vi "(Sub) Save.vi"(0 "IN Path":path, 2 "C Limit / Voltage":dbl[](array[numeric]), 3 "G1. V":dbl, 4 "G2. V":dbl, 5 "error in (no error)":errorcluster caption="에러 입력(에러 없음)", 6 "State":enum16{"Open", "Header Make", "Save", "Close"}(ring), 7 "G3. V":dbl, 8 "G1. Info":string, 9 "G1. A":dbl, 10 "G2. Info":string, 11 "G2. A":dbl, 12 "G3. Info":string, 13 "G3. A":dbl) -> (14 "Save Path":path, 19 "error out":errorcluster caption="에러 출력")   [LabVIEW 2017]
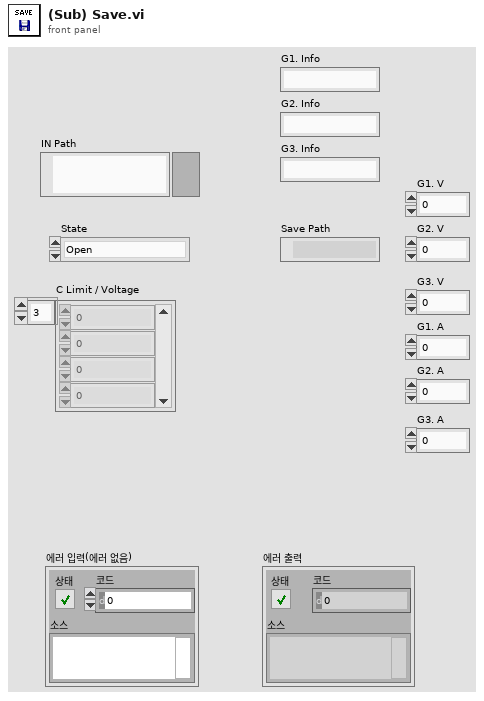
[diagram p1: front panel]
types:
  T1 = enum16{"open", "replace", "create", "open or create", "replace or create", "replace or create with confirmation"}
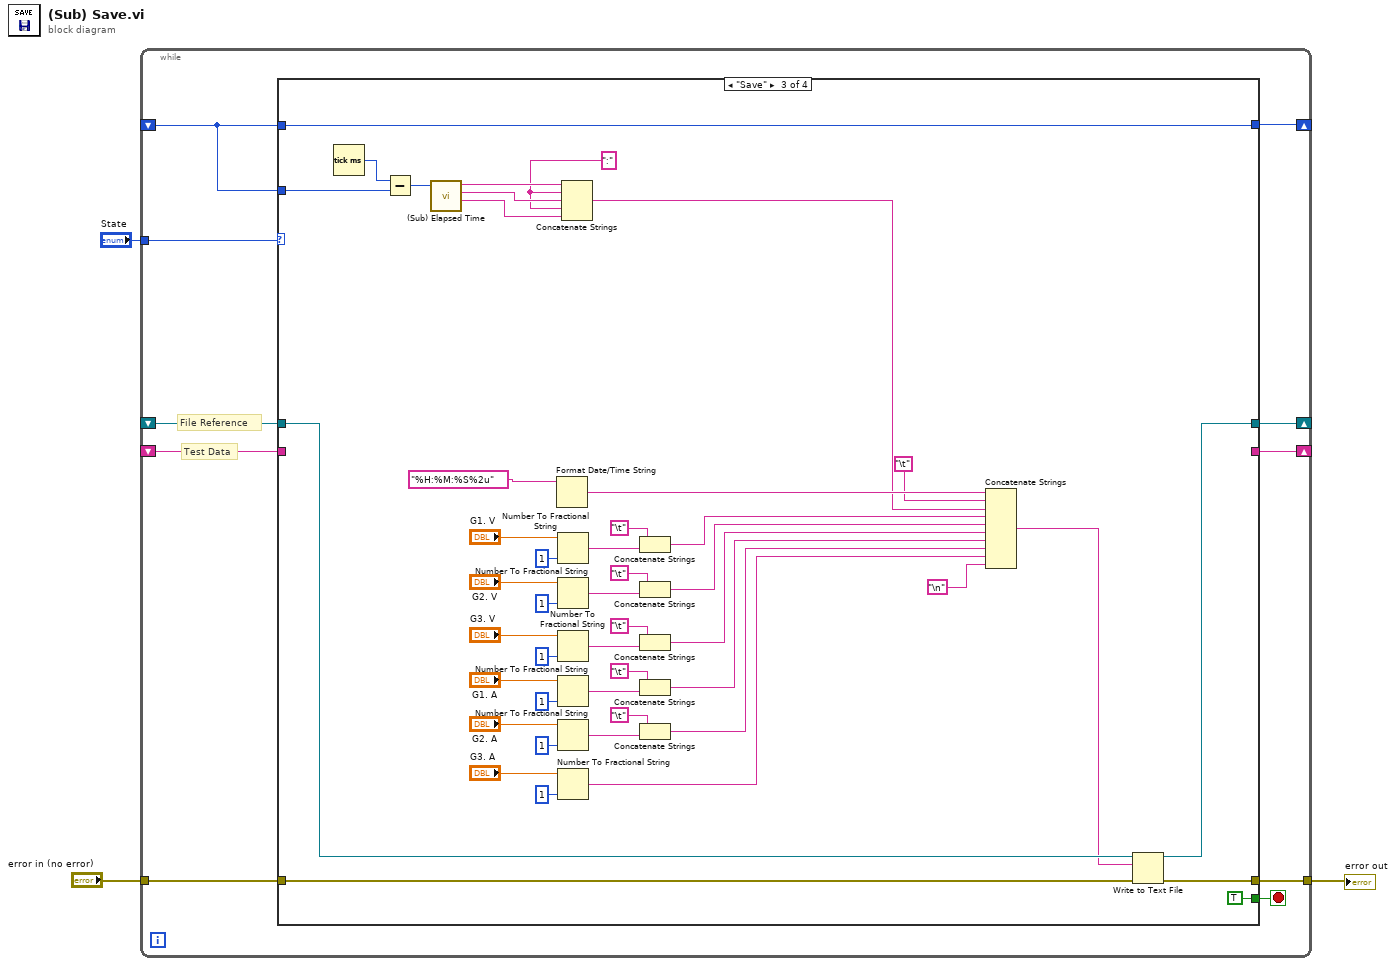
[diagram p0: block diagram]
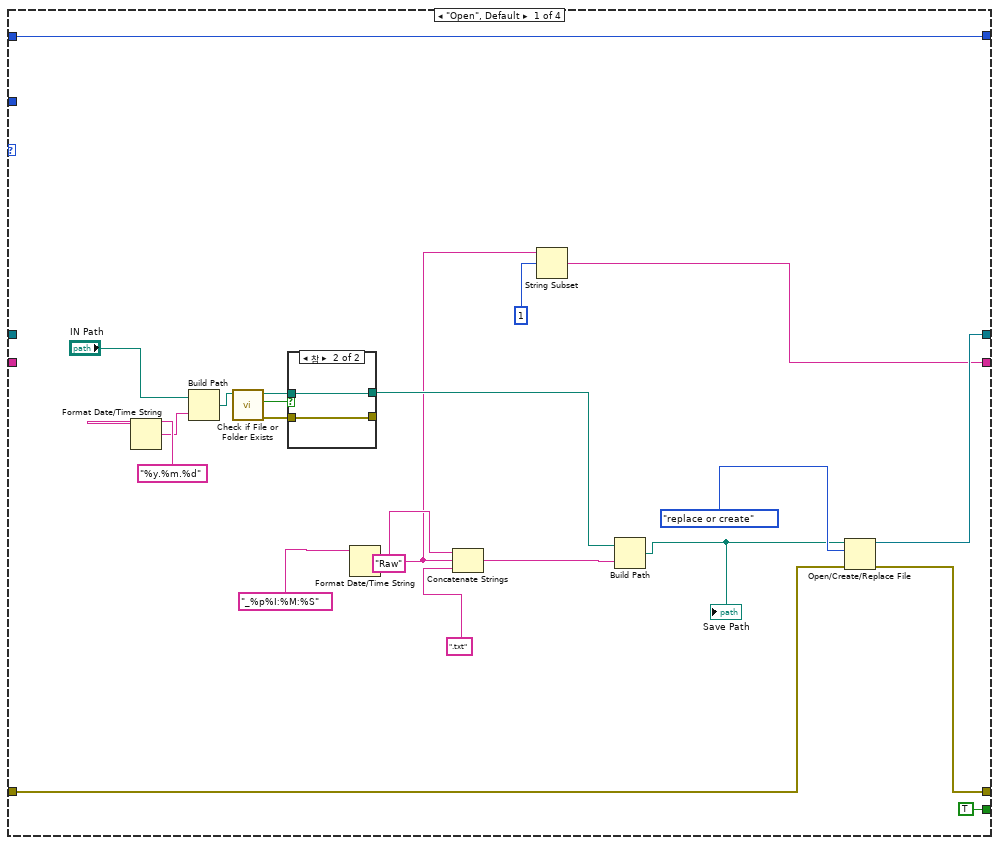
[diagram p2: hidden frame]
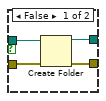
[diagram p3: hidden frame]
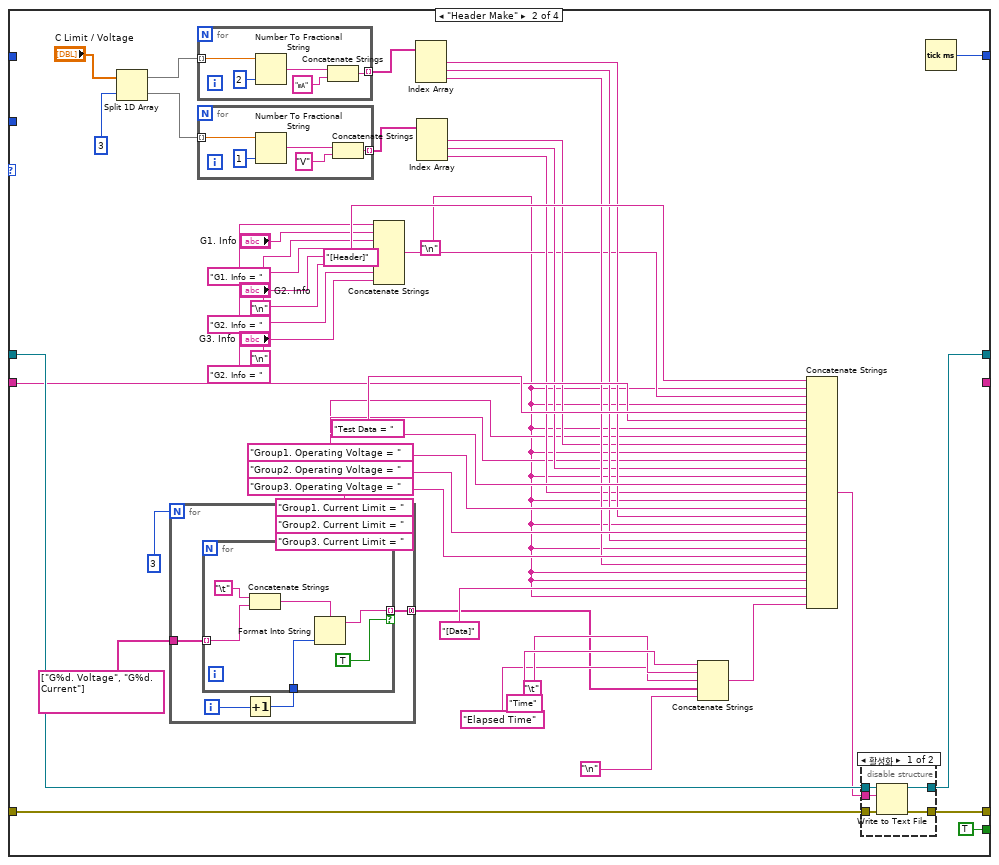
[diagram p4: hidden frame]
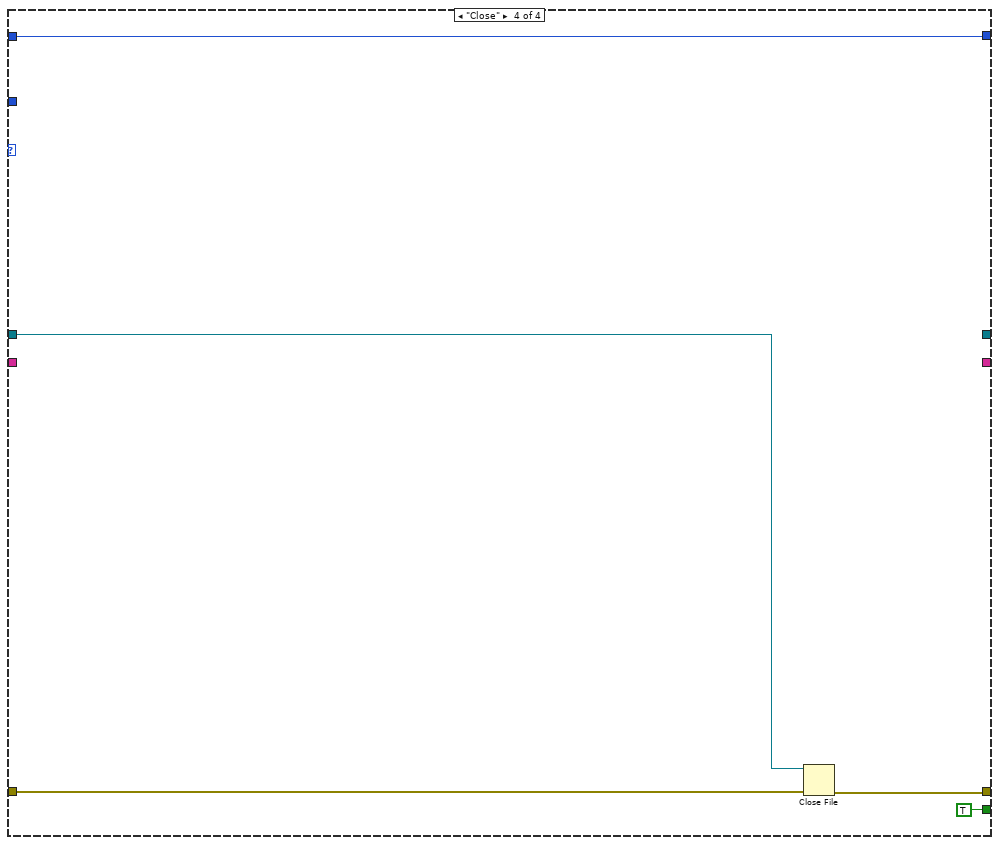
[diagram p6: hidden frame]
diagram:
  n1 = while {
    tunnel: [w10] -> w2
    tunnel: "error in (no error)" -> [w13]
    shift-right: [w11] -> _
    shift-left: _ -> [w12]
    shift-right: [w9] -> _
    shift-left: _ -> [w8]
    shift-right: [w6] -> _
    shift-left: _ -> [w5]
    tunnel: "State" -> [w4]
    stop <- w7 stop-if-true
    # "Test Data"
    # "File Reference"
    n2 = case shown="\"Save\"" w4 {
      tunnel: w13 -> [w30 w88 w160 w164]
      tunnel: w12 -> [_ w81 w157 w163]
      tunnel: [w33 w80 w154 _] -> w11
      tunnel: [w32 w87 w159 w165] -> w10
      tunnel: [w14 _ _ _] -> w9
      tunnel: w8 -> [_ w78 _ _]
      tunnel: [TRUE TRUE TRUE TRUE] -> w7
      tunnel: [w27 w77 w145 w161] -> w6
      tunnel: w5 -> [_ _ w146 _]
      tunnel: w5 -> [w27 _ w145 w161]
      frame "Open", Default {
        n3 = Format Date/Time String(time format string (%c)="%y.%m.%d" ("시간 포맷 문자열 (%c)")) -> (date/time string=w25:string)  [unwired: 2 in]
        n4 = Build Path(base path="IN Path", name or relative path=w25) -> (appended path=w24:path)
        n5 = call <vilib>:"Check if File or Folder Exists.vi"("path"=w24) -> ("error out"=w21:errorcluster, "file or folder exists?"=w23:bool, "dup path"=w22:path)  [unwired: 8 in]
        n6 = case shown="참" w23 {
          tunnel: w22 -> [w39 w41]
          tunnel: w21 -> [w38 w40]
          tunnel: [w37 w41] -> w20
          tunnel: [w36 w40] -> _
          frame False {
            n7 = Create Folder(path (use dialog)=w39, error in=w38) -> (created path=w37:path, error out=w36:errorcluster)  [unwired: 1 in, 1 out]
          }
          frame True {
          }
        }
        n8 = Format Date/Time String(time format string (%c)="_%p%Iː%Mː%S" ("시간 포맷 문자열 (%c)")) -> (date/time string=w16:string)  [unwired: 2 in]
        n9 = Concatenate Strings("Raw" ("문자열"), w16, ".txt") -> (w31:string)
        n10 = String Subset(string=w16, offset (0)=1 ("오프셋(0)")) -> (substring=w14:string)  [unwired: 1 in]
        n11 = Build Path(base path=w20, name or relative path=w31) -> (appended path=w28:path)
        "Save Path" <- w28
        n12 = Open/Create/Replace File(file path (use dialog)=w28, error in=w30, operation (0:open)=T1."replace or create" ("동작(0:open)")) -> (refnum out=w33:refnum<file>, error out=w32:errorcluster)  [unwired: 3 in, 1 out]
      }
      frame "Header Make" {
        w42 = "\n"
        n13 = Split 1D Array(array="C Limit / Voltage", index=3 ("인덱스")) -> (first subarray=w64:dbl[], second subarray=w63:dbl[])
        n14 = for {
          N: 3 -> [_]
          tunnel: [w107] -> w71 mode=concatenating
          tunnel: string[] ["G%d. Voltage", "G%d. Current"] -> [w106]
          i -> [w105]
          n15 = Increment(x=w105) -> (x+1=w104:i32)
          n16 = for {
            tunnel: [w113] -> w107 mode=indexing if=TRUE
            tunnel: w106 -> [w110] mode=indexing
            tunnel: w104 -> [w109]
            n17 = Concatenate Strings("\t", w110) -> (w111:string)
            n18 = Format Into String(format string=w111, w109) -> (resulting string=w113:string)  [unwired: 2 in, 1 out]
          }
        }
        n19 = for {
          tunnel: w64 -> [w97] mode=indexing
          tunnel: [w94] -> w62 mode=indexing
          n20 = Number To Fractional String(number=w97, precision (6)=i16 2 ("정밀도(6)")) -> (F-format string=w96:string)  [unwired: 2 in]
          n21 = Concatenate Strings(w96, "㎃") -> (w94:string)
        }
        n22 = for {
          tunnel: w63 -> [w92] mode=indexing
          tunnel: [w89] -> w58 mode=indexing
          n23 = Number To Fractional String(number=w92, precision (6)=i16 1 ("정밀도(6)")) -> (F-format string=w90:string)  [unwired: 2 in]
          n24 = Concatenate Strings(w90, "V") -> (w89:string)
        }
        n25 = Concatenate Strings("G1. Info = ", "G1. Info", "\n", "G2. Info = ", "G2. Info", "\n", "G2. Info = ", "G3. Info") -> (w44:string)
        n26 = Index Array(array=w62) -> (element #1=w61:string, element #2=w60:string, element #3=w59:string)  [unwired: 3 in]
        n27 = Index Array(array=w58) -> (element #1=w54:string, element #2=w56:string, element #3=w57:string)  [unwired: 3 in]
        n28 = Concatenate Strings("Time", "\t", "Elapsed Time", w71, "\n") -> (w70:string)
        n29 = Concatenate Strings("[Header]", w42, w44, w42, "Test Data = ", w78, w42, "Group1. Operating Voltage = ", w54, w42, "Group2. Operating Voltage = ", w56, w42, "Group3. Operating Voltage = ", w57, w42, "Group1. Current Limit = ", w61, w42, "Group2. Current Limit = ", w60, w42, "Group3. Current Limit = ", w59, w42, w42, "[Data]", w42, w70) -> (w79:string)
        n30 = disable-structure shown="활성화" {
          disable-tunnel: w88 -> [w103 _]
          disable-tunnel: [w102 _] -> w87
          disable-tunnel: w81 -> [w101 _]
          disable-tunnel: [w100 _] -> w80
          disable-tunnel: w79 -> [w99 _]
          frame Enabled {
            n31 = Write to Text File(file (use dialog)=w101, text=w99, error in=w103) -> (refnum out=w100:refnum<file>, error out=w102:errorcluster)  [unwired: 1 in, 1 out]
          }
          frame Disabled {
          }
        }
        n32 = Tick Count (ms)() -> (millisecond timer value=w77:u32)
      }
      frame "Save" {
        w148 = "ː"
        n33 = Tick Count (ms)() -> (millisecond timer value=w153:u32)
        n34 = Subtract(x=w153, y=w146) -> (x-y=w152:u32)
        n35 = call "(Sub) Elapsed Time.vi"("In ms"=w152) -> ("S"=w149:string, "M"=w150:string, "H"=w151:string)  [unwired: 7 in, 1 out]
        n36 = Format Date/Time String(time format string (%c)="%Hː%Mː%S%2u" ("시간 포맷 문자열 (%c)")) -> (date/time string=w156:string)  [unwired: 2 in]
        n37 = Number To Fractional String(number="G1. V", precision (6)=i16 1 ("정밀도(6)")) -> (F-format string=w141:string)  [unwired: 2 in]
        n38 = Number To Fractional String(number="G2. V", precision (6)=i16 1 ("정밀도(6)")) -> (F-format string=w138:string)  [unwired: 2 in]
        n39 = Number To Fractional String(number="G3. V", precision (6)=i16 1 ("정밀도(6)")) -> (F-format string=w133:string)  [unwired: 2 in]
        n40 = Number To Fractional String(number="G1. A", precision (6)=i16 1 ("정밀도(6)")) -> (F-format string=w130:string)  [unwired: 2 in]
        n41 = Number To Fractional String(number="G2. A", precision (6)=i16 1 ("정밀도(6)")) -> (F-format string=w125:string)  [unwired: 2 in]
        n42 = Number To Fractional String(number="G3. A", precision (6)=i16 1 ("정밀도(6)")) -> (F-format string=w114:string)  [unwired: 2 in]
        n43 = Concatenate Strings(w151, w148, w150, w148, w149) -> (w147:string)
        n44 = Concatenate Strings("\t", w141) -> (w120:string)
        n45 = Concatenate Strings("\t", w138) -> (w119:string)
        n46 = Concatenate Strings("\t", w133) -> (w118:string)
        n47 = Concatenate Strings("\t", w130) -> (w117:string)
        n48 = Concatenate Strings("\t", w125) -> (w116:string)
        n49 = Concatenate Strings(w156, "\t", w147, w120, w119, w118, w117, w116, w114, "\n") -> (w155:string)
        n50 = Write to Text File(file (use dialog)=w157, text=w155, error in=w160) -> (refnum out=w154:refnum<file>, error out=w159:errorcluster)  [unwired: 1 in, 1 out]
      }
      frame "Close" {
        n51 = Close File(refnum=w163, error in=w164) -> (error out=w165:errorcluster)  [unwired: 1 out]
      }
    }
  }
  "error out" <- w2
